vi "Configure Servo.vi"(8 "error in":errorcluster, 11 "tCRD in":refnum<class "Open Path CRD.lvclass">) -> (0 "error out":errorcluster, 3 "tCRD out":refnum<class "Open Path CRD.lvclass">)   [LabVIEW 2015, in "Open Path CRD.lvclass"]
uses:
  Open Path CRD.lvclass
  Switch/Servo Switch.lvclass
  Reusable/Session APIs/File Access/Config Data/Config Data.lvclass
  Reusable/Instrument/Instrument.lvclass/Instrument.ctl
  Reusable/Session APIs/File Access/Config Data/Config Data.lvclass/Config Data.ctl
  Switch/Servo Switch.lvclass/Servo Switch.ctl
  Reusable/Switch/Switch.lvclass/Switch.ctl
  Open Path CRD.lvclass/Open Path CRD.ctl
  Reusable/Instrument/Read Cfg Session.vi
  Reusable/Session APIs/File Access/Config Data/Accessors/Read Ref.vi
  Switch/Write High Time.vi
  Switch/Write Low Time.vi
  Reusable/Switch/Write LastSwitch.vi
  <vilib>/Utility/config.llb/Read Key (Boolean).vi
  <vilib>/Utility/config.llb/Read Key (Double).vi
  <vilib>/Utility/config.llb/Read Key (I32).vi
  Reusable/Switch/Write maxElapseTime.vi
  <userlib>/_Session Fwk/Session - Root.lvclass
  <vilib>/Utility/config.llb/NI_LVConfig.lvlib
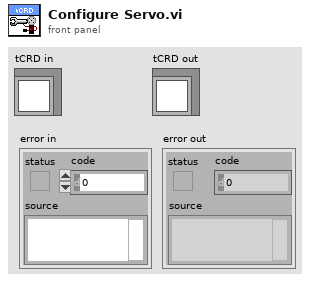
[diagram p1: front panel]
types:
  T1 = typedef "Session - Root.lvclass/Session Handle.ctl" = refnum<data-value>
  T2 = typedef "NI_LVConfig.lvlib/Config Data RefNum.ctl" = refnum<k1>
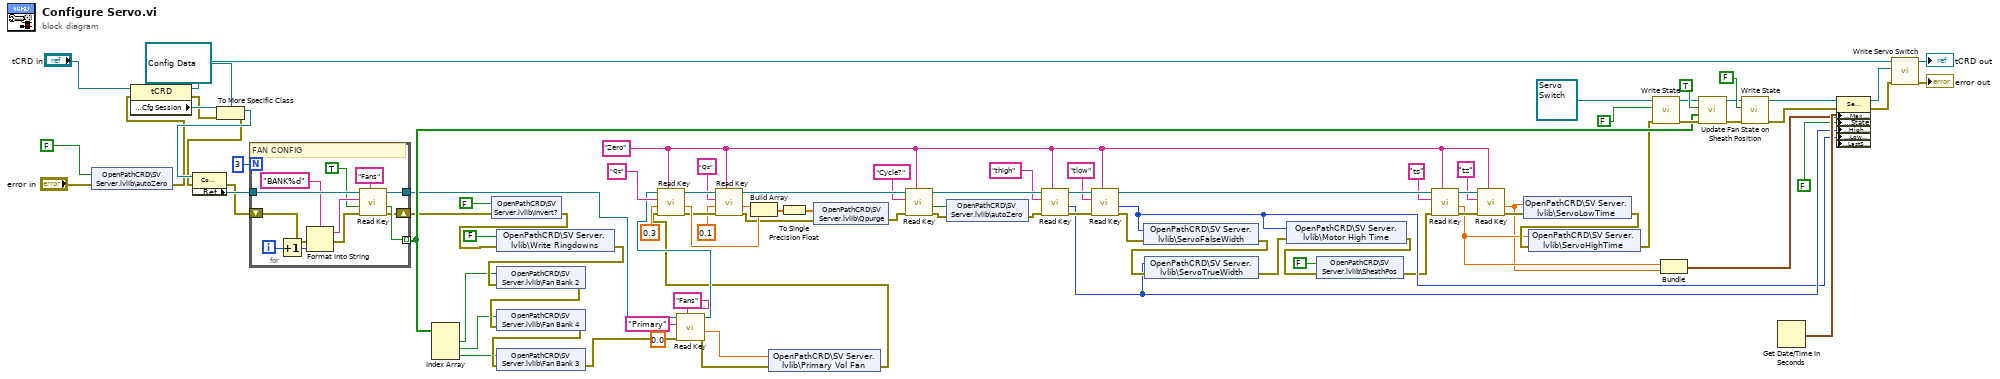
[diagram p0: block diagram]
diagram:
  w55 = "Zero" ("section")
  n1 = shared-variable "OpenPathCRD\\SV Server.lvlib\\autoZero"(FALSE ("autoZero"), error in="error in") -> (error out=w2:errorcluster)
  n2 = property class="tCRD"(reference="tCRD in", error in=w2) -> (reference out=w7:refnum<class "Open Path CRD.lvclass">, error out=w3:errorcluster, "Accessors:Cfg Session"=w6:T1)
  n3 = To More Specific Class(target class=refnum<data-value> refnum, reference=w6, error in=w3) -> (specific class reference=w4:refnum<data-value>, error out=w1:errorcluster)
  n4 = property class="Config Data"(reference=w4, error in=w1) -> (error out=w22:errorcluster, "Accessors:Ref"=w23:T2)  [unwired: 1 out]
  n5 = for {
    N: 3 -> [_]
    tunnel: w23 -> [w103]
    tunnel: [w97] -> w25 mode=indexing
    tunnel: [w95] -> w17
    shift-right: [w93] -> w20
    shift-left: w22 -> [w92]
    i -> [w101]
    # "FAN CONFIG"
    n6 = Increment(x=w101) -> (x+1=w100:i32)
    n7 = Format Into String(format string="BANK%d", error in=w92, w100) -> (resulting string=w98:string, error out=w94:errorcluster)  [unwired: 1 in]
    n8 = call-poly <vilib>:"Read Key.vi"("section"="Fans", "error in (no error)"=w94, "default value"=TRUE, "key"=w98, "refnum"=w103) -> ("error out"=w93:errorcluster, "value"=w97:bool, "refnum out"=w95:T2)  [unwired: 3 in, 1 out]
  }
  n9 = Index Array(array=w25) -> (element #1=w35:bool, element #2=w34:bool, element #3=w33:bool)  [unwired: 3 in]
  n10 = shared-variable "OpenPathCRD\\SV Server.lvlib\\Invert?"(FALSE ("Invert?"), error in=w20) -> (error out=w21:errorcluster)
  n11 = shared-variable "OpenPathCRD\\SV Server.lvlib\\Write Ringdowns"(FALSE ("Write Ringdowns"), error in=w21) -> (error out=w39:errorcluster)
  n12 = shared-variable "OpenPathCRD\\SV Server.lvlib\\Fan Bank 2"(w35, error in=w39) -> (error out=w38:errorcluster)
  n13 = shared-variable "OpenPathCRD\\SV Server.lvlib\\Fan Bank 4"(w34, error in=w38) -> (error out=w37:errorcluster)
  n14 = shared-variable "OpenPathCRD\\SV Server.lvlib\\Fan Bank 3"(w33, error in=w37) -> (error out=w13:errorcluster)
  n15 = call-poly <vilib>:"Read Key.vi"("section"="Fans", "error in (no error)"=w13, "default value"=0.0, "key"="Primary", "refnum"=w17) -> ("error out"=w10:errorcluster, "value"=w11:dbl, "refnum out"=w16:T2)  [unwired: 3 in, 1 out]
  n16 = shared-variable "OpenPathCRD\\SV Server.lvlib\\Primary Vol Fan"(w11, error in=w10) -> (error out=w9:errorcluster)
  n17 = call-poly <vilib>:"Read Key.vi"("section"=w55, "error in (no error)"=w9, "default value"=0.3, "key"="Qz", "refnum"=w16) -> ("error out"=w76:errorcluster, "value"=w77:dbl, "refnum out"=w81:T2)  [unwired: 3 in, 1 out]
  n18 = call-poly <vilib>:"Read Key.vi"("section"=w55, "error in (no error)"=w76, "default value"=0.1, "key"="Qs", "refnum"=w81) -> ("error out"=w75:errorcluster, "value"=w78:dbl, "refnum out"=w72:T2)  [unwired: 3 in, 1 out]
  n19 = Build Array(w78, w77) -> (w74:dbl[])
  n20 = To Single Precision Float(number=w74) -> (single precision float=w73:sgl[])
  n21 = shared-variable "OpenPathCRD\\SV Server.lvlib\\Qpurge"(w73, error in=w75) -> (error out=w71:errorcluster)
  n22 = call-poly <vilib>:"Read Key.vi"("section"=w55, "error in (no error)"=w71, "key"="Cycle?", "refnum"=w72) -> ("error out"=w68:errorcluster, "value"=w69:bool, "refnum out"=w67:T2)  [unwired: 4 in, 1 out]
  n23 = shared-variable "OpenPathCRD\\SV Server.lvlib\\autoZero"(w69, error in=w68) -> (error out=w66:errorcluster)
  n24 = call-poly <vilib>:"Read Key.vi"("section"=w55, "error in (no error)"=w66, "key"="thigh", "refnum"=w67) -> ("error out"=w64:errorcluster, "value"=w51:i32, "refnum out"=w65:T2)  [unwired: 4 in, 1 out]
  n25 = call-poly <vilib>:"Read Key.vi"("section"=w55, "error in (no error)"=w64, "key"="tlow", "refnum"=w65) -> ("error out"=w60:errorcluster, "value"=w50:i32, "refnum out"=w61:T2)  [unwired: 4 in, 1 out]
  n26 = shared-variable "OpenPathCRD\\SV Server.lvlib\\ServoFalseWidth"(w50, error in=w60) -> (error out=w58:errorcluster)
  n27 = shared-variable "OpenPathCRD\\SV Server.lvlib\\ServoTrueWidth"(w51, error in=w58) -> (error out=w46:errorcluster)
  n28 = shared-variable "OpenPathCRD\\SV Server.lvlib\\Motor High Time"(w50, error in=w46) -> (error out=w45:errorcluster)
  n29 = shared-variable "OpenPathCRD\\SV Server.lvlib\\SheathPos"(FALSE ("SheathPos"), error in=w45) -> (error out=w44:errorcluster)
  n30 = call-poly <vilib>:"Read Key.vi"("section"=w55, "error in (no error)"=w44, "key"="ts", "refnum"=w61) -> ("error out"=w56:errorcluster, "value"=w49:dbl, "refnum out"=w57:T2)  [unwired: 4 in, 1 out]
  n31 = call-poly <vilib>:"Read Key.vi"("section"=w55, "error in (no error)"=w56, "key"="tz", "refnum"=w57) -> ("error out"=w53:errorcluster, "value"=w48:dbl)  [unwired: 4 in, 2 out]
  n32 = shared-variable "OpenPathCRD\\SV Server.lvlib\\ServoLowTime"(w48, error in=w53) -> (error out=w52:errorcluster)
  n33 = shared-variable "OpenPathCRD\\SV Server.lvlib\\ServoHighTime"(w49, error in=w52) -> (error out=w19:errorcluster)
  n34 = call-dynamic "Write State.vi"("error in"=w19, "State"=FALSE ("SheathPos"), "Switch in"=refnum<class "Servo Switch.lvclass"> refnum ("Servo Switch in")) -> ("error out"=w26:errorcluster, "Switch out"=w28:refnum<class "Servo Switch.lvclass">)  [unwired: 7 in]
  n35 = Bundle("value"=w49, "value"=w48) -> (w47:cluster{"value":dbl, "value":dbl})  [unwired: 1 in]
  n36 = call "Update Fan State on Sheath Position.vi"("error in"=w26, "Init Fan Pos"=w25, "Init?"=TRUE, "Servo Switch in"=w28) -> ("error out"=w18:errorcluster, "Servo Switch out"=w24:refnum<class "Servo Switch.lvclass">)  [unwired: 6 in]
  n37 = call-dynamic "Write State.vi"("error in"=w18, "State"=FALSE ("SheathPos"), "Switch in"=w24) -> ("error out"=w89:errorcluster, "Switch out"=w88:refnum<class "Servo Switch.lvclass">)  [unwired: 7 in]
  n38 = Get Date/Time In Seconds() -> (seconds since 1Jan1904=w91:timestamp)
  n39 = property class="Servo Switch"(reference=w88, error in=w89, "Data Access:Max Elapsed Time"=w47, "Data Access:State"=FALSE ("State"), "Accessors:High Time"=w51, "Accessors:Low Time"=w50, "Accessors:LastSwitch"=w91) -> (reference out=w86:refnum<class "Servo Switch.lvclass">, error out=w83:errorcluster)
  n40 = call "Write Servo Switch.vi"("error in (no error)"=w83, "Servo Switch"=w86, "tCRD in"=w7) -> ("error out"=→"error out":errorcluster, "tCRD out"=→"tCRD out":refnum<class "Open Path CRD.lvclass">)  [unwired: 7 in]
